vi "T_step_initial_T_control.vi"(11 "Current T step Setpoint":dbl) -> ()   [LabVIEW 2019]
uses:
  Monitors/Utility/Monitor Communication/LS370/LS370-Control.ctl
  Global/Global Variables/global.vi
  Global/Global Variables/Data_Display_global.vi
  Instrument_Setup.vi
  Monitors/Utility/Monitor Communication/sub-vis/LS370_Open_Queue.vi
panel:
  out "Numeric 3":dbl format="%#_13g"
  out "Numeric 2":dbl format="%#_13g"
  out "XY Graph":T1(graph)
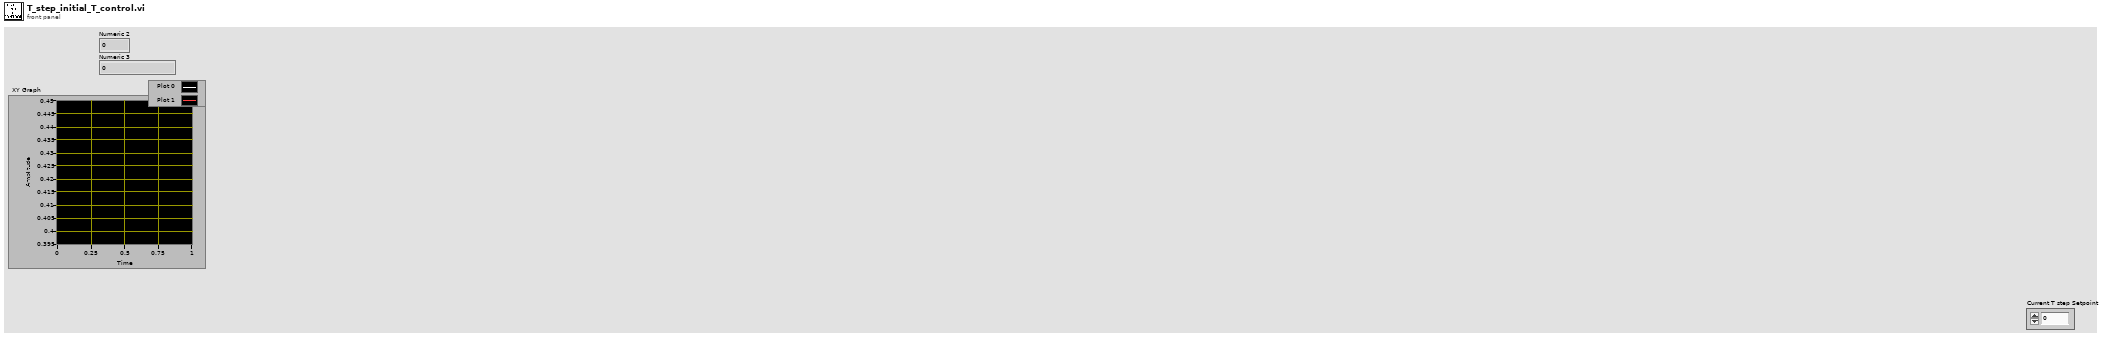
[diagram p1: front panel]
types:
  T1 = cluster{"Plot1":dbl[], "Best Linear Fit":dbl[]}[]
  T2 = typedef "LS370-Control.ctl" = cluster{"Disable Heater":bool, "Activate Tsweep":bool, "Update Lakeshores":bool, "Setpoint - Manual":dbl, "Rate (K/min)":dbl, "Sorb Power (mW)":dbl, "Still Power (mW)":dbl, "Sorb Heater":bool, "Still Heater":bool, "Set Temperature Sweep Main":bool}
  T3 = typedef "LS372-Cluster.ctl" = cluster{"Activate Tsweep":bool, "Setpoint - Manual":dbl, "Rate (K/min)":dbl, "Update Lakeshores":bool, "Still Heater":bool, "Still Power (mW)":dbl, "Manual Heater":bool, "Manual Heater  (mW) ":dbl, "Heater Range":dbl, "P (Gain)":dbl, "I (Reset)":dbl, "D (Rate)":dbl, "Heater Power (mW)":dbl, "MC Thermometer":u16, "MC Temperature":dbl, "LS372-T1":dbl, "LS372 -T2":dbl, "LS372-R1 ":dbl, "LS372-R2":dbl, "LS372-T3":dbl, "LS372-T4":dbl, "LS372-R3 ":dbl, "LS372-R4 \n\n\n\n":dbl, "LS372-T5":dbl, "LS372-T6":dbl, "LS372-R5":dbl, "LS372-R6 ":dbl, "Still Power ist":dbl, "Set Temperatur Sweep main":bool, "Setpoint ist":dbl, "Disable Heater":bool}
  T4 = typedef "Ls372-Control.ctl" = cluster{"Activate Tsweep":bool, "Setpoint - Manual":dbl, "Rate (K/min)":dbl, "Update Lakeshores":bool, "Still Heater":bool, "Still Power (mW)":dbl, "Manual Heater":bool, "Manual Heater  (mW) ":dbl, "MC Thermometer":u16, "Set Temperature Sweeep main":bool, "Disable Heater":bool}
  T5 = typedef "P9P14-TCluster.ctl" = cluster{"Setpoint":dbl, "Rate":dbl, "Chanel 1":dbl, "Approach":u16, "Set":bool, "Temperature\nStatus":i32, "Autoshutdown":bool}
  T6 = typedef "P9P14-TCluster-Control.ctl" = cluster{"Setpoint":dbl, "Rate":dbl, "Approach":u16, "Set":bool, "Autoshutdown":bool}
  T7 = typedef "ITC503Monitor-Cluster.ctl" = cluster{"Temperatur (K)":dbl, "Setpoint (K)":dbl, "Rate (K/min)":dbl, "Heater (%)":dbl, "NV (%)":dbl, "Heater Manual":bool, "NV Manual":bool, "Go to Set":bool, "Heater SP":dbl, "Valid?":bool, "Set Heater SP":bool, "Set NV SP":bool, "Heater (%) Display":dbl, "NV (%) Display":dbl, "NV Setpoint":dbl, "Change Heater Status":bool, "Change NV Status":bool, "Sample 3":dbl, "Sample 2":dbl, "Sweep-State":bool, "Set Auto PID":bool, "Auto PID":bool, "Stopp":bool, "Setpoint-Sweep":dbl, "Sample 1":dbl, "Control Channel":bool, "Channel 1":bool, "Channel 2":bool, "Channel 3":bool}
  T8 = typedef "ITC503_control.ctl" = cluster{"Setpoint (K)":dbl, "Rate (K/min)":dbl, "Go to Set":bool, "Set Heater SP":bool, "Set NV SP":bool, "Change Heater Status":bool, "Change NV Status":bool, "Set Auto PID":bool, "Stopp":bool, "Control Channel":bool, "Heater SP":dbl, "NV Setpoint":dbl}
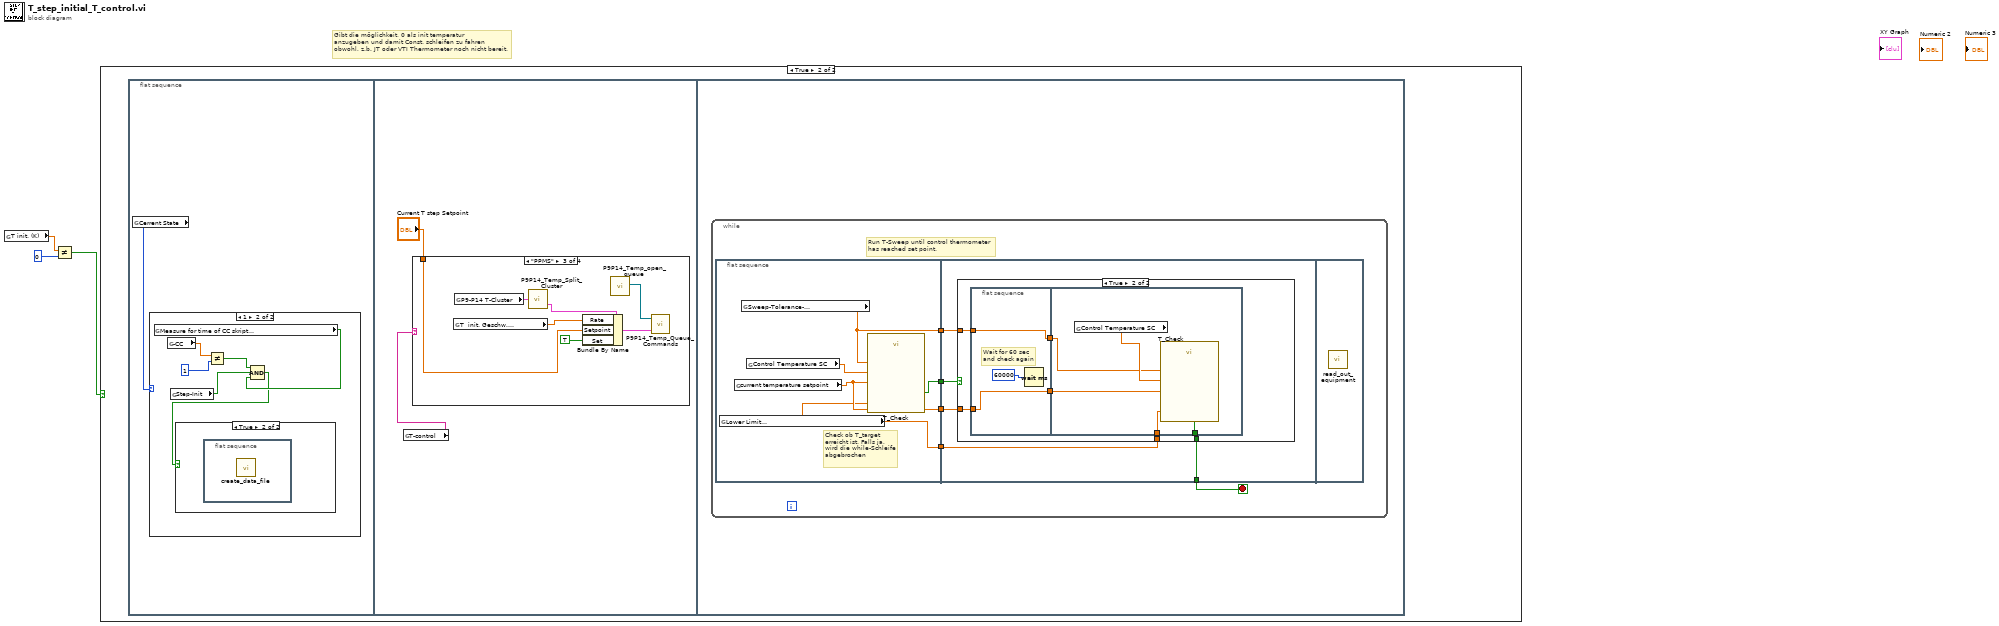
[diagram p0: block diagram]
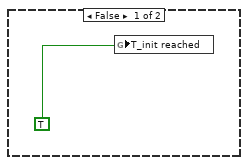
[diagram p2: hidden frame]
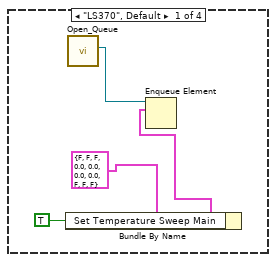
[diagram p5: hidden frame]
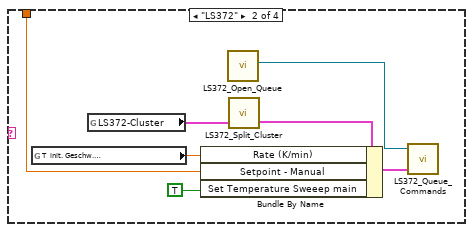
[diagram p6: hidden frame]
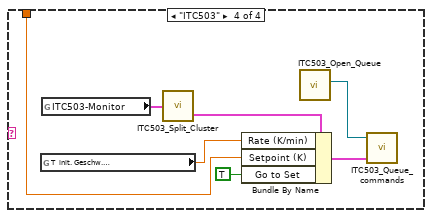
[diagram p7: hidden frame]
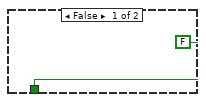
[diagram p8: hidden frame]
diagram:
  # "Gibt die möglichkeit, 0 als init temperatur \nanzugeben und damit Const. schleifen zu fahren\nobwohl, z.b. JT oder VTI Thermometer noch nicht bereit."
  n1 = global read "global.vi" "T init. (K)"() -> (w3:dbl)
  n2 = Not Equal?(x=w3, y=0) -> (x != y?=w1:bool)
  n3 = case shown="True" w1 {
    frame False {
      n4 = global write "Data_Display_global.vi" "T_init reached"(TRUE) -> ()
    }
    frame True {
      n5 = flat-sequence {
        frame #0 {
          n6 = global read "global.vi" "Cerrent State"() -> (w5:i32)
          n7 = case shown="1" w5 {
            frame 0, Default {
            }
            frame 1 {
              n8 = global read "Instrument_Setup.vi" "Measure for time of CC skript\nat each field step point"() -> (w7:bool)
              n9 = global read "global.vi" "-CC"() -> (w11:dbl)
              n10 = global read "global.vi" "Step-Init"() -> (w8:bool)
              n11 = Not Equal?(x=w11, y=1) -> (x != y?=w9:bool)
              n12 = Compound Arithmetic op=AND(w9, w8, w7) -> (w6:bool)
              n13 = case shown="True" w6 {
                frame False {
                }
                frame True {
                  n14 = flat-sequence {
                    frame #0 {
                      n15 = call "create_data_file.vi"() -> ()  [unwired: 3 in]
                    }
                  }
                }
              }
            }
          }
        }
        frame #1 {
          n16 = global read "Instrument_Setup.vi" "T-control"() -> (w13:string)
          n17 = case shown="\"PPMS\"" w13 {
            tunnel: "Current T step Setpoint" -> [_ w18 w25 w32]
            frame "LS370", Default {
              n18 = Bundle By Name(cluster=T2 {"Disable Heater"=FALSE, "Activate Tsweep"=FALSE, "Update Lakeshores"=FALSE, "Setpoint - Manual"=0.0, "Rate (K/min)"=0.0, "Sorb Power (mW)"=0.0, "Still Power (mW)"=0.0, "Sorb Heater"=FALSE, "Still Heater"=FALSE, "Set Temperature Sweep Main"=FALSE} ("JT-Cluster"), "Set Temperature Sweep Main"=TRUE) -> (w14:T2)
              n19 = call-poly "Open_Queue.vi"() -> ("queue out"=w17:refnum<queue>)  [unwired: 10 in, 1 out]
              n20 = Enqueue Element(queue=w17, element=w14) -> ()  [unwired: 2 in, 3 out]
            }
            frame "LS372" {
              n21 = global read "global.vi" "T  init. Geschw. \n(K/min)"() -> (w21:dbl)
              n22 = global read "Data_Display_global.vi" "LS372-Cluster"() -> (w24:T3)
              n23 = call "LS372_Open_Queue.vi"() -> ("queue out"=w20:refnum<queue>)  [unwired: 10 in, 1 out]
              n24 = call "LS372_Split_Cluster.vi"("LS372-Cluster"=w24) -> ("LS372-Control"=w23:T4)  [unwired: 1 out]
              n25 = Bundle By Name(cluster=w23, "Rate (K/min)"=w21, "Setpoint - Manual"=w18, "Set Temperature Sweeep main"=TRUE) -> (w19:T4)
              n26 = call "LS372_Queue_Commands.vi"("LS372-Control"=w19, "Queue"=w20) -> ()  [unwired: 1 in, 1 out]
            }
            frame "PPMS" {
              n27 = global read "global.vi" "T  init. Geschw. \n(K/min)"() -> (w31:dbl)
              n28 = global read "Data_Display_global.vi" "P9-P14 T-Cluster"() -> (w26:T5)
              n29 = call "P9P14_Temp_Split_Cluster.vi"("P9-P14 T-Cluster"=w26) -> ("P9-P14 T-Cluster -Control"=w27:T6)  [unwired: 1 out]
              n30 = Bundle By Name(cluster=w27, "Rate"=w31, "Setpoint"=w25, "Set"=TRUE) -> (w29:T6)
              n31 = call "P9P14_Temp_open_queue.vi"() -> ("queue out"=w30:refnum<queue>)  [unwired: 10 in, 1 out]
              n32 = call "P9P14_Temp_Queue_Commands.vi"("P9-P14 T-Cluster -Control"=w29, "Queue"=w30) -> ()  [unwired: 1 in, 1 out]
            }
            frame "ITC503" {
              n33 = global read "global.vi" "T  init. Geschw. \n(K/min)"() -> (w38:dbl)
              n34 = global read "Data_Display_global.vi" "ITC503-Monitor"() -> (w36:T7)
              n35 = call "ITC503_Split_Cluster.vi"("ITC503-Monitor"=w36) -> ("ITC503-Control"=w35:T8)  [unwired: 1 out]
              n36 = Bundle By Name(cluster=w35, "Rate (K/min)"=w38, "Setpoint (K)"=w32, "Go to Set"=TRUE) -> (w34:T8)
              n37 = call "ITC503_Open_Queue.vi"() -> ("queue out"=w37:refnum<queue>)  [unwired: 10 in, 1 out]
              n38 = call "ITC503_Queue_commands.vi"("ITC503-Control"=w34, "ITC503 Queue"=w37) -> ()  [unwired: 1 in, 1 out]
            }
          }
        }
        frame #2 {
          n39 = while {
            stop <- w42 stop-if-true
            # "Run T-Sweep until control thermometer\nhas reached set point."
            n40 = flat-sequence {
              tunnel: [w47] -> w43
              tunnel: [w45] -> w41
              tunnel: [w46] -> w40
              tunnel: [w44] -> w39
              tunnel: w43 -> [w53]
              tunnel: [w52] -> w42
              tunnel: w41 -> [w51]
              tunnel: w40 -> [w50]
              tunnel: w39 -> [w49]
              frame #0 {
                # "Check ob T_target\nerreicht ist. Falls ja,\nwird die while-Schleife\nabgebrochen"
                n41 = global read "Instrument_Setup.vi" "Lower Limit\nSweep-Tolerance-\nTemperature (K)"() -> (w44:dbl)
                n42 = global read "Data_Display_global.vi" "current temperature setpoint"() -> (w45:dbl)
                n43 = global read "Instrument_Setup.vi" "Sweep-Tolerance-\nTemperature (%)"() -> (w46:dbl)
                n44 = global read "Data_Display_global.vi" "Control Temperature SC"() -> (w48:dbl)
                n45 = call "T_Check.vi"("Lower Limit Sweep\nTolerance (K)"=w44, "T_target (K)"=w45, "Sweep\nTolerance %"=w46, "T_in"=w48) -> ("= T target"=w47:bool)
              }
              frame #1 {
                n46 = case shown="True" w53 {
                  tunnel: [FALSE w60] -> w52
                  tunnel: w51 -> [_ w59]
                  tunnel: w50 -> [_ w56]
                  tunnel: w49 -> [_ w55]
                  frame False {
                  }
                  frame True {
                    n47 = flat-sequence {
                      tunnel: w59 -> [w62]
                      tunnel: [w62] -> w58
                      tunnel: [w61] -> w57
                      tunnel: w56 -> [w61]
                      tunnel: [w68] -> w60
                      tunnel: w58 -> [w66]
                      tunnel: w57 -> [w65]
                      tunnel: w55 -> [w64]
                      frame #0 {
                        # "Wait for 60 sec\nand check again"
                        n48 = Wait (ms)(milliseconds to wait=60000) -> ()  [unwired: 1 out]
                      }
                      frame #1 {
                        n49 = global read "Data_Display_global.vi" "Control Temperature SC"() -> (w67:dbl)
                        n50 = call "T_Check.vi"("Lower Limit Sweep\nTolerance (K)"=w64, "T_target (K)"=w66, "Sweep\nTolerance %"=w65, "T_in"=w67) -> ("= T target"=w68:bool)
                      }
                    }
                  }
                }
              }
              frame #2 {
                n51 = call "read_out_equipment.vi"() -> ()  [unwired: 1 in]
              }
            }
          }
        }
      }
    }
  }
